vi "RSZVB Set Frequency RF Conversion Factor.vi"(7 "Denominator (1)":i32=1, 8 "error in (no error)":errorcluster {"code" format="%.0x"}, 9 "Numerator (1)":i32=1, 10 "Channel (1)":i32=1, 11 "VISA resource name":refnum<visa-resource-name>) -> (0 "error out":errorcluster {"code" format="%.0x"}, 3 "VISA resource name out":refnum<visa-resource-name>)   [LabVIEW 2011]
doc: "This VI sets the frequency conversion factors for the RF signal.\n\nNotes:\n\nThe frequency conversion factors for vector mixer measurements (options R&S ZVA-K5) must be equal to 1.\n\nRemote-control command(s):\n[SENSe<Ch>:]FREQuency:CONVersion:MIXer:RFMultiplier <numerator>,<denominator>"
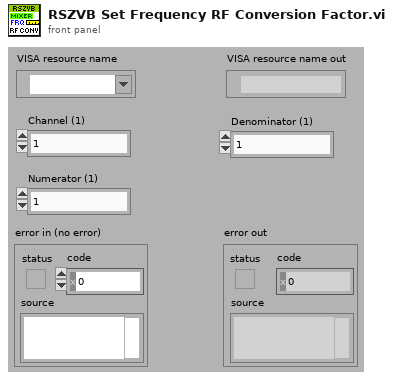
[diagram p1: front panel]
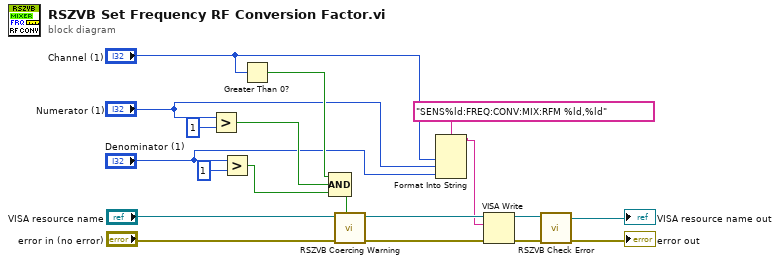
[diagram p0: block diagram]
diagram:
  n1 = Greater?(x="Numerator (1)", y=1) -> (0:w4:bool)
  n2 = Greater?(x="Denominator (1)", y=1) -> (0:w3:bool)
  n3 = Greater Than 0?(x="Channel (1)") -> (x > 0?=w12:bool)
  n4 = Compound Arithmetic op=AND(w12, w4, w3) -> (w15:bool)
  n5 = call "RSZVB Coercing Warning.vi"("In Range?"=w15, "error in (no error)"="error in (no error)", "VISA session"="VISA resource name") -> ("error out"=w18:errorcluster, "dup VISA session"=w19:refnum<visa-resource-name>)  [unwired: 7 in]
  n6 = Format Into String(format string="SENS%ld:FREQ:CONV:MIX:RFM %ld,%ld", "Channel (1)", "Numerator (1)", "Denominator (1)") -> (resulting string=w13:string)  [unwired: 2 in, 1 out]
  n7 = VISA Write(VISA resource name=w19, write buffer=w13, error in (no error)=w18) -> (VISA resource name out=w16:refnum<visa-resource-name>, error out=w17:errorcluster)  [unwired: 1 out]
  n8 = call "RSZVB Check Error.vi"("error in (no error)"=w17, "VISA session"=w16) -> ("error out"=→"error out":errorcluster, "dup VISA session"=→"VISA resource name out":refnum<visa-resource-name>)  [unwired: 8 in]
